vi "live view D04.vi"() -> ()   [LabVIEW 2019, in "D04.lvlib"]
uses:
  D04.lvlib
  <vilib>/userDefined/High Color/IMAQdx.ctl
  <vilib>/vision/Image Controls.llb/IMAQ Image.ctl
  <vilib>/measure/mamon.llb/Trigger Detection for 1 Channel.vi
  <vilib>/measure/NI_MAPro.lvlib
  Calibration Lib.lvlib
  database.lvlib
  <vilib>/vision/driver/NI_Vision_Acquisition_Software.lvlib
panel:
  out "Error out":errorcluster
  in  "Save Button":bool
  in  "Calib IMQ Num":u16(ring) items=["First IMQ", "Second IMQ", "Third IMQ"]
  in  "Verify Calibration1 D04":bool caption="capture grab"
  in  "snapshot":bool
  out "error prj03":errorcluster
  in  "Verify Calibration D04":bool caption="capture grab"
  in  "Close":bool
  in  "Method 2 save D04":bool caption="capture grab"
  in  "Method 1 Save D04":bool caption="Saving txt"
  out "Average Result":string="Average Result"
  out ">18  A":dbl(slide)=1.0 caption=">18 mm" scale=0.0..100.0
  out "16-18  A":dbl(slide)=1.0 caption="16-18 mm" scale=0.0..100.0
  out "14-16  A":dbl(slide)=1.0 caption="14-16 mm" scale=0.0..100.0
  out "12.5-14 A":dbl(slide)=1.0 caption="12.5-14 mm" scale=0.0..100.0
  out "10-12.5  A":dbl(slide)=1.0 caption="10-12.5 mm" scale=0.0..100.0 scale format="%#_4f"
  out "8-10  A":dbl(slide)=1.0 caption="8-10 mm" scale=0.0..100.0
  out "6.3-8  A":dbl(slide)=1.0 caption="6.3-8 mm" scale=0.0..100.0
  out "<6.3  A":dbl(slide)=1.0 caption="<6.3 mm" scale=0.0..100.0
  out "Live Result":string="Live Result"
  out ">18  L":dbl(slide)=1.0 caption=">18 mm" scale=0.0..100.0
  out "Live View":T1(plugin-control) caption="Disc 26"
  out "16-18  L":dbl(slide)=1.0 caption="16-18 mm" scale=0.0..100.0
  out "14-16  L":dbl(slide)=1.0 caption="14-16 mm" scale=0.0..100.0
  out "12.5-14 L":dbl(slide)=1.0 caption="12.5-14 mm" scale=0.0..100.0
  out "10-12.5  L":dbl(slide)=1.0 caption="10-12.5 mm" scale=0.0..100.0 scale format="%#_4f"
  out "8-10  L":dbl(slide)=1.0 caption="8-10 mm" scale=0.0..100.0
  out "6.3-8  L":dbl(slide)=1.0 caption="6.3-8 mm" scale=0.0..100.0
  out "<6.3  L":dbl(slide)=1.0 caption="<6.3 mm" scale=0.0..100.0
  out "disc name":string="Live Info Disc 04"
  out "dsgs":string="DSGS"
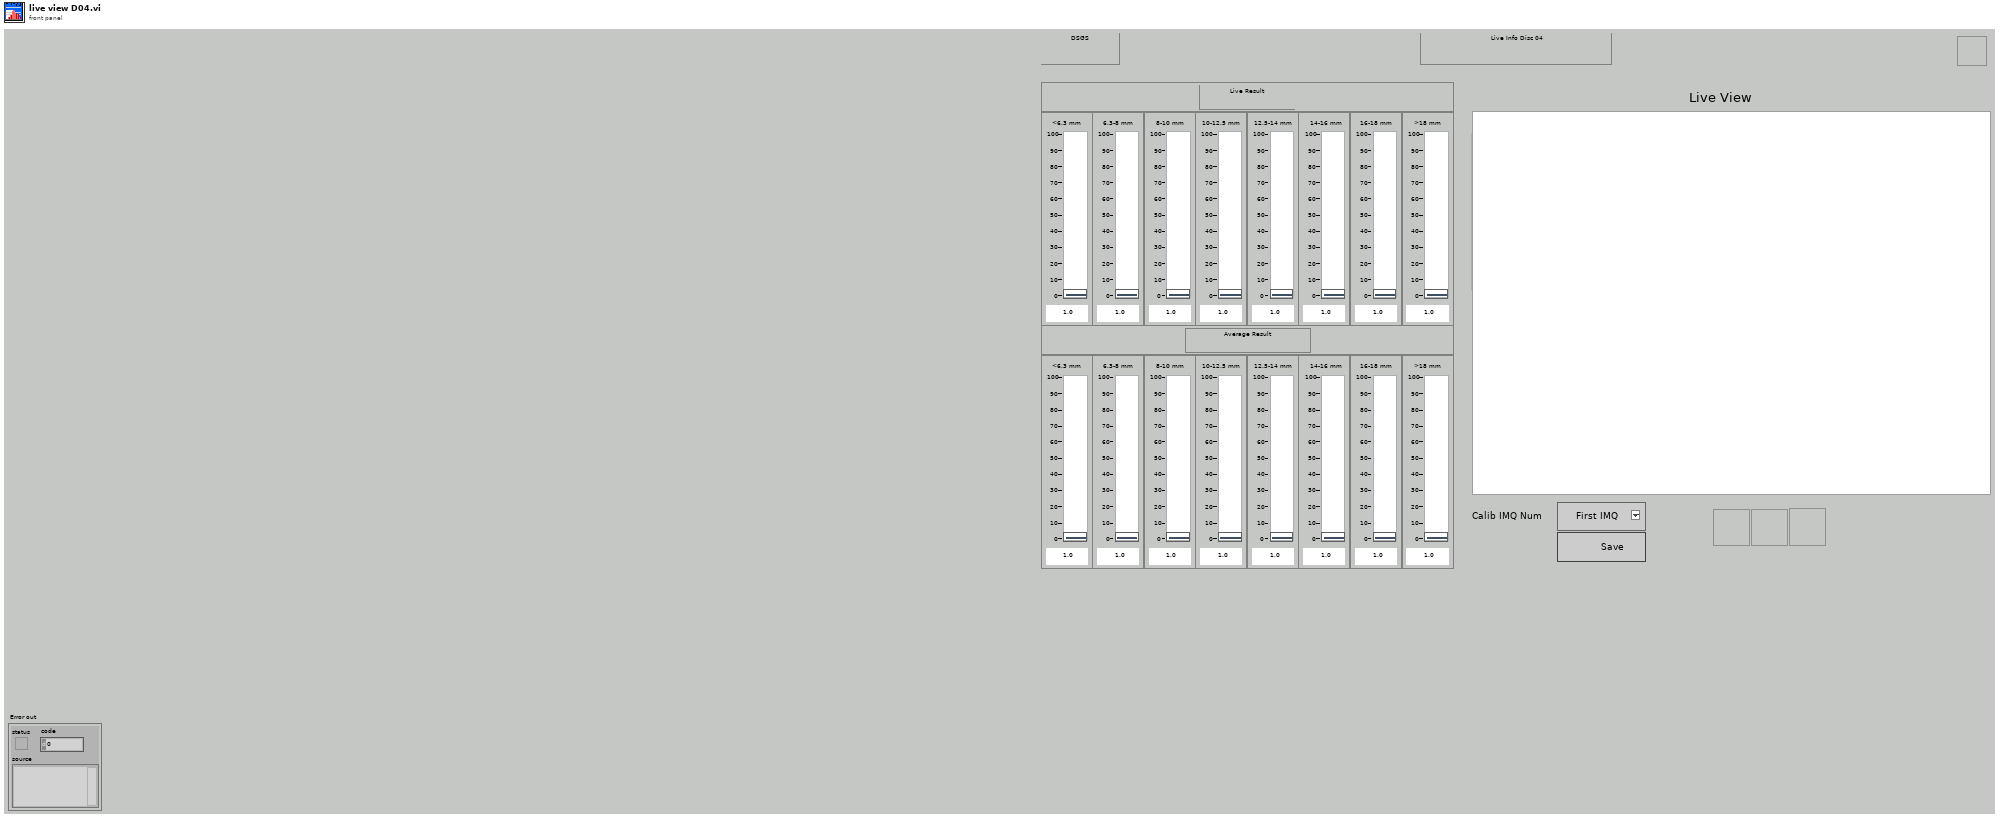
[diagram p1: front panel]
types:
  T1 = typedef "IMAQ Image.ctl" = refnum<image>
  T2 = typedef "IMAQdx.ctl" = refnum<k21>
  T3 = enum8{"Enabled", "Disabled", "Disabled and Grayed Out"}
  T4 = cluster{"date/time string":string, "date/time string":string, string, "Value":dbl, "Value":dbl, "Value":dbl, "Value":dbl, "Value":dbl, "Value":dbl, "Value":dbl, "Value":dbl}
  T5 = cluster{"date/time string":string, "date/time string":string, "time format string (%c)":string, "spreadsheet string":string, "spreadsheet string":string}
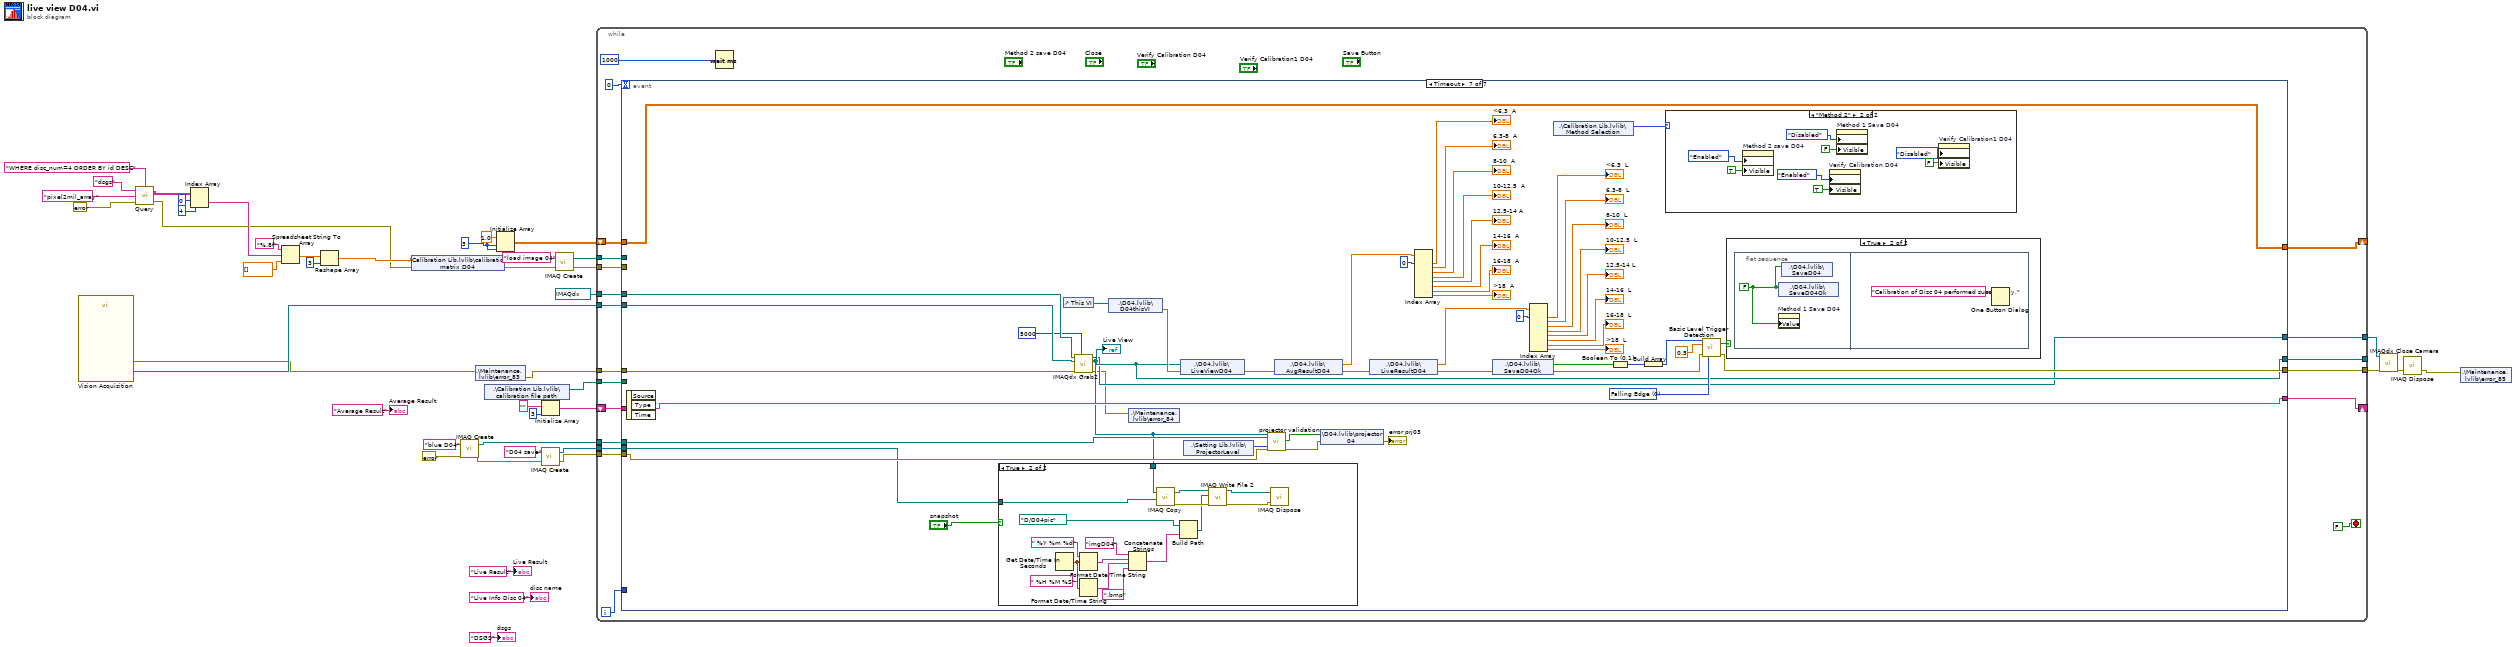
[diagram p0: block diagram]
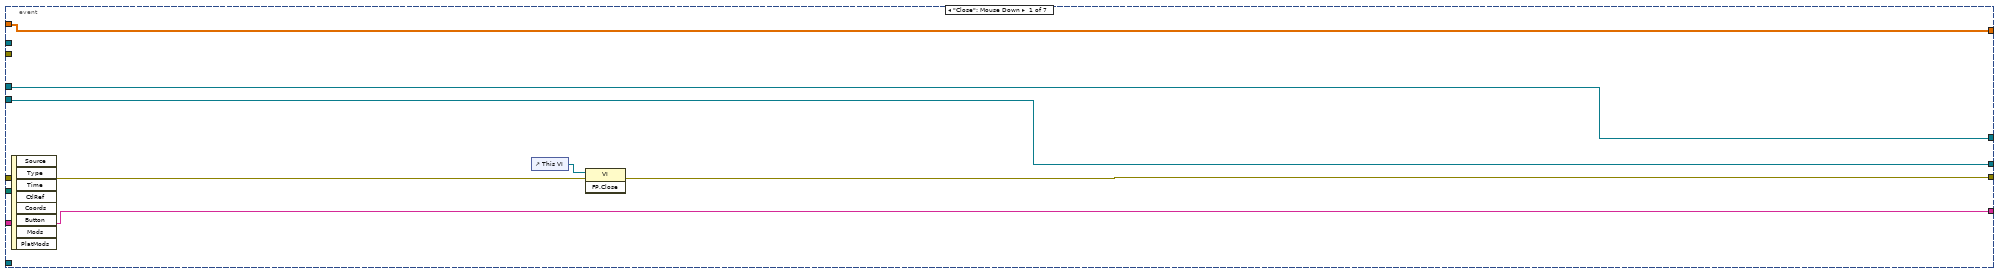
[diagram p2: hidden frame]
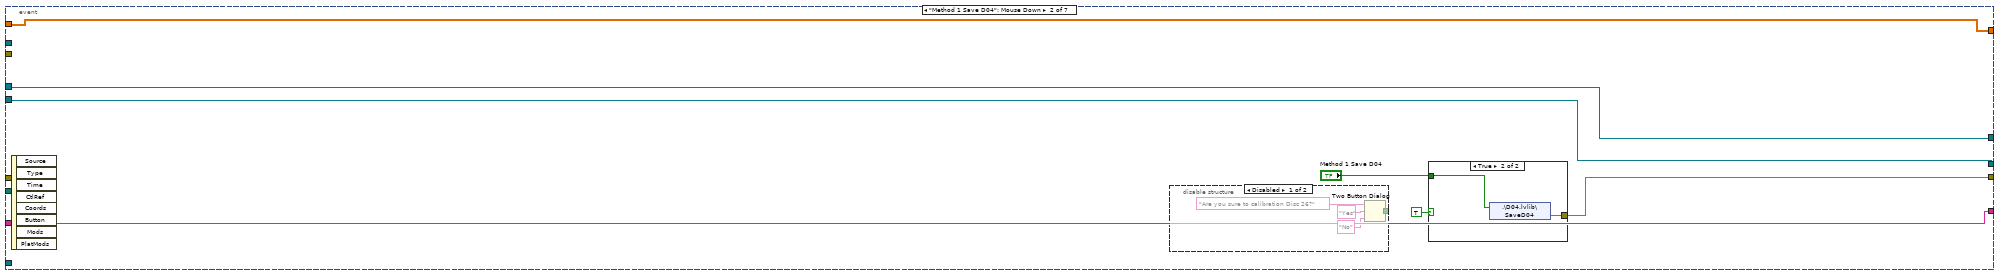
[diagram p3: hidden frame]
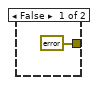
[diagram p5: hidden frame]
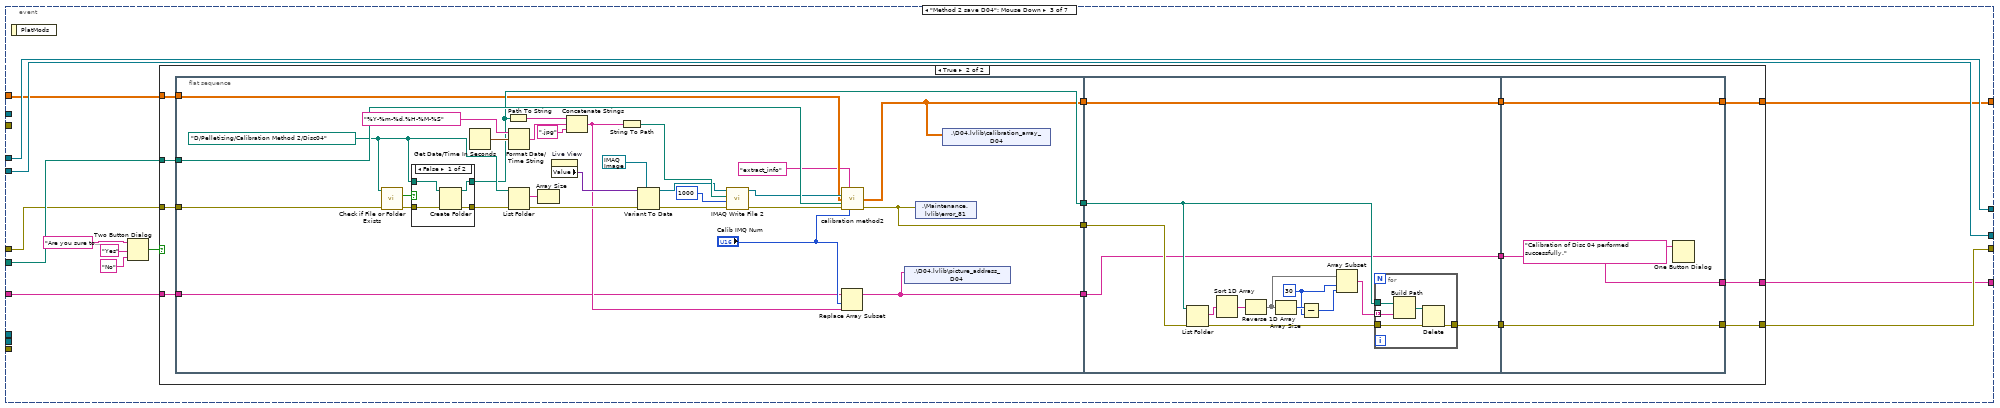
[diagram p6: hidden frame]
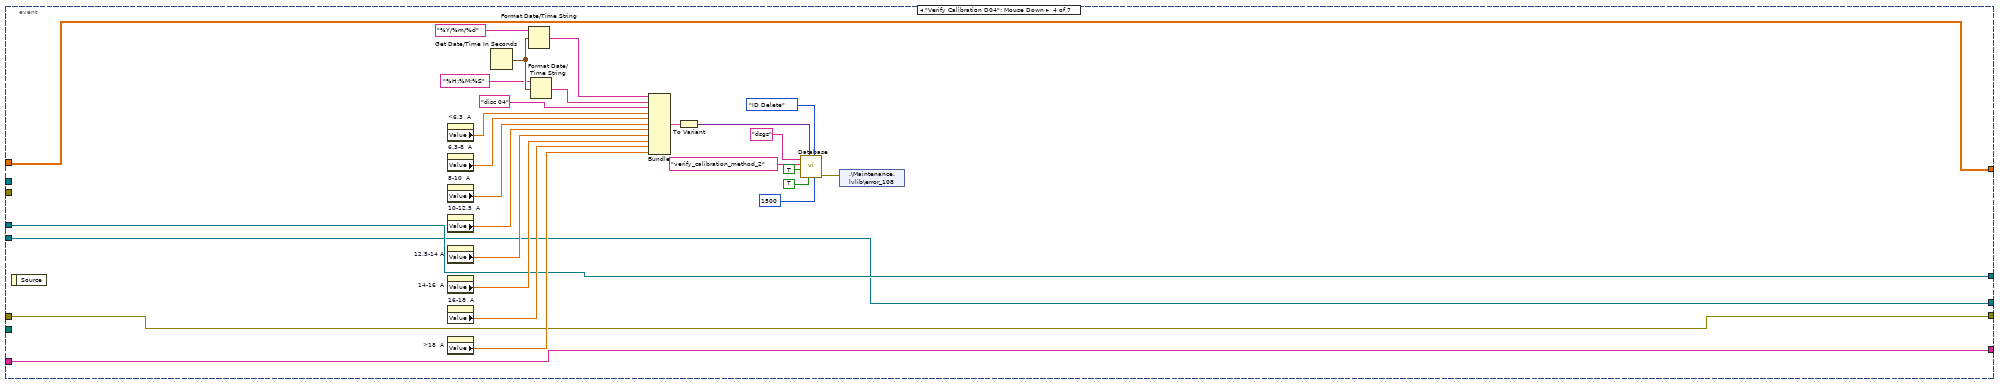
[diagram p9: hidden frame]
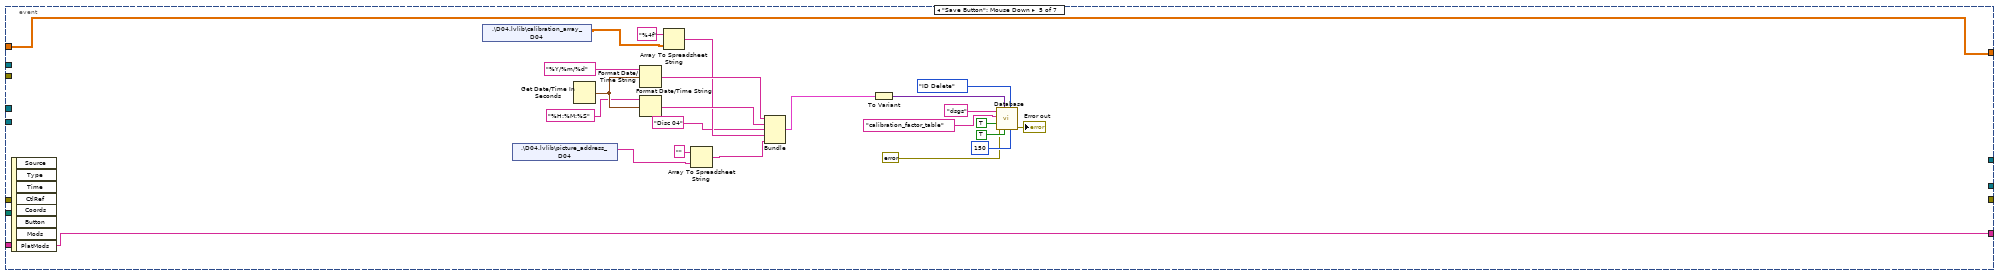
[diagram p10: hidden frame]
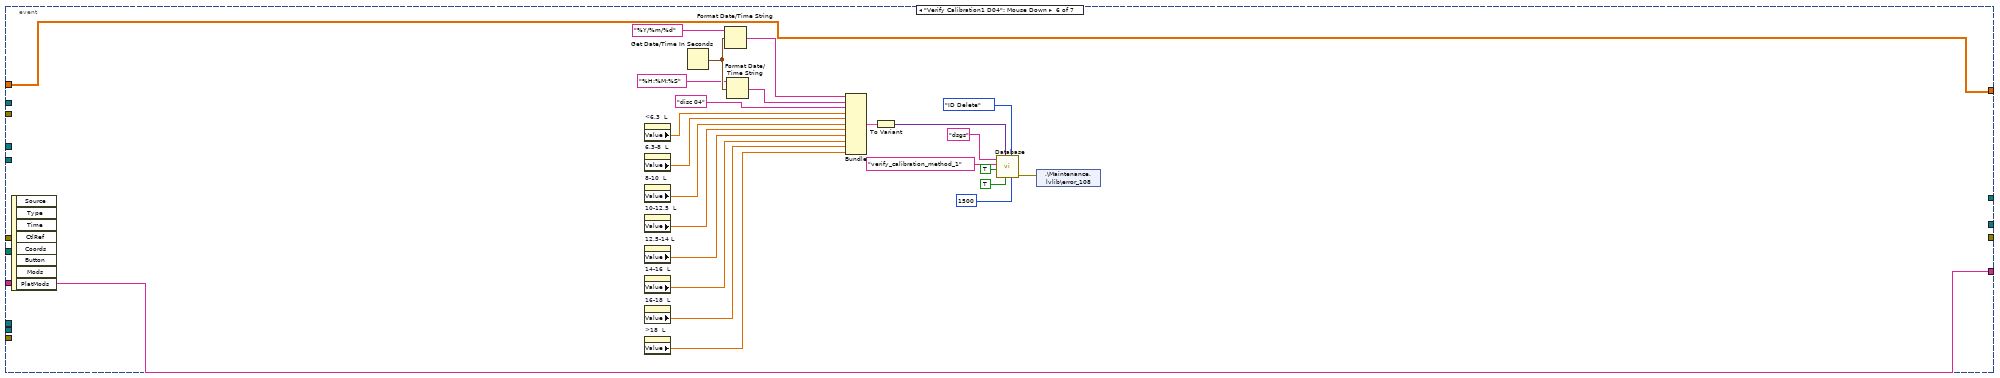
[diagram p11: hidden frame]
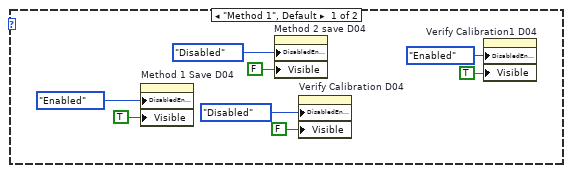
[diagram p13: hidden frame]
diagram:
  w13 = 3 ("dimension size")
  n1 = call "Vision Acquisition"() -> ("Image Out"=w2:T1, "error out"=w1:errorcluster)  [unwired: 25 in, 1 out]
  n2 = call "Query.vi"("Condition"="WHERE disc_num=4 ORDER BY id DESC", "Error in"=errorcluster {"status"=FALSE, "code"=0, "source"=""}, "Table Name"="pixel2mil_array", "Connection Name"="dsgs") -> ("Error out"=w5:errorcluster, "data"=w8:string[][])
  n3 = Index Array(array=w8, index (row)=0, index (col)=4 ("disabled index (col)")) -> (element=w6:string)
  n4 = Spreadsheet String To Array(format string="%.8f", spreadsheet string=w6, array type (2D Dbl)=sgl[] []) -> (array=w26:sgl[])  [unwired: 1 in]
  n5 = Reshape Array(w26, 3 ("dimension size")) -> (w23:sgl[])
  n6 = shared-variable ".\\Calibration Lib.lvlib\\calibration matrix D04"(w23, error in=w5) -> (error out=w22:errorcluster)
  n7 = call "IMAQ Create"("Image Name"="blue D04", "error in (no error)"=errorcluster {"status"=FALSE, "code"=0, "source"=""}) -> ("New Image"=w20:T1, "error out"=w18:errorcluster)  [unwired: 3 in]
  n8 = shared-variable ".\\Maintenance.lvlib\\error_83"(w1) -> (error out=w35:errorcluster)  [unwired: 1 in]
  n9 = shared-variable ".\\Calibration Lib.lvlib\\calibration file path"() -> (w36:path)  [unwired: 1 in, 1 out]
  n10 = Initialize Array(1.0 ("element"), w13, w13) -> (w12:dbl[][])
  n11 = call "IMAQ Create"("Image Name"="D04 save", "error in (no error)"=w18) -> ("New Image"=w15:T1, "error out"=w17:errorcluster)  [unwired: 3 in]
  n12 = Initialize Array("", 3 ("dimension size")) -> (w9:string[])
  n13 = call "IMAQ Create"("Image Name"="load image 04", "error in (no error)"=w22) -> ("New Image"=w32:T1, "error out"=w33:errorcluster)  [unwired: 3 in]
  n14 = while {
    tunnel: w36 -> [w62]
    tunnel: w35 -> [w61]
    tunnel: w2 -> [w59]
    tunnel: [w58] -> w40
    tunnel: [w57] -> _
    tunnel: T2 "disc01" ("Session In") -> [w56]
    tunnel: [w55] -> w37
    tunnel: w33 -> [w54]
    tunnel: w32 -> [w53]
    tunnel: w20 -> [w52]
    tunnel: w17 -> [w51]
    tunnel: w15 -> [w50]
    shift-right: [w47] -> _
    shift-left: w12 -> [w48]
    shift-right: [w45] -> _
    shift-left: w9 -> [w46]
    i -> [w49]
    stop <- FALSE stop-if-true
    n15 = event shown="[6] Timeout" {
      selector: _ -> [_ _ _ _ _ _ _]
      dyn-events: _ -> [_ _ _ _ _ _ _]
      timeout: 0 -> [_ _ _ _ _ _ _]
      tunnel: w62 -> [_ _ w98 _ _ _ _]
      tunnel: [w70 w78 w94 w180 _ _ w269] -> w58
      tunnel: w61 -> [w69 _ w97 w180 _ _ w254]
      tunnel: w59 -> [w68 w77 w96 w178 _ _ w253]
      tunnel: [w68 w77 w96 w178 _ _ w257] -> w57
      tunnel: w56 -> [w67 w76 w95 w179 _ _ w256]
      tunnel: [w67 w76 w95 w179 _ _ w255] -> w55
      tunnel: w54 -> [_ _ _ _ _ _ _]
      tunnel: w53 -> [_ _ _ _ _ _ _]
      tunnel: w52 -> [_ _ _ _ _ _ w267]
      tunnel: w51 -> [_ _ _ _ _ _ w263]
      tunnel: w50 -> [_ _ _ _ _ _ w260]
      tunnel: w49 -> [_ _ _ _ _ _ _]
      tunnel: w48 -> [w66 w73 w89 w175 w204 w227 w259]
      tunnel: [w66 w73 w88 w175 w204 w227 w259] -> w47
      tunnel: w46 -> [w65 w72 w87 w174 w203 w226 w258]
      tunnel: [w65 w72 w86 w174 w203 w226 w258] -> w45
      event "Close": Mouse Down {
        n16 = event-data() -> ()  [unwired: 1 in, 8 out]
        n17 = control-ref of="This VI"() -> (w71:refnum<vi>)
        n18 = invoke class="VI" method="FP.Close"(reference=w71, error in=w69) -> (error out=w70:errorcluster)  [unwired: 1 in, 2 out]
      }
      event "Method 1 Save D04": Mouse Down {
        n19 = event-data() -> ()  [unwired: 1 in, 8 out]
        n20 = disable-structure shown="Disabled" {
          disable-tunnel: [w79 _] -> _
          frame Disabled {
            n21 = Two Button Dialog(message="Are you sure to calibration Disc 26?", 1:"No" ("F button name (\"Cancel\")"), 2:"Yes" ("T button name (\"OK\")")) -> (T button?=w79:bool)
          }
          frame Enabled {
          }
        }
        n22 = case shown="True" TRUE {
          tunnel: [errorcluster {"status"=FALSE, "code"=0, "source"=""} ("error IO") w85] -> w78
          tunnel: "Method 1 Save D04" -> [_ w84]
          frame False {
          }
          frame True {
            n23 = shared-variable ".\\D04.lvlib\\SaveD04"(w84) -> (error out=w85:errorcluster)  [unwired: 1 in]
          }
        }
      }
      event "Method 2 save D04": Mouse Down {
        n24 = event-data() -> ()  [unwired: 1 in, 1 out]
        n25 = Two Button Dialog(message="Are you sure to calibration Disc 26?", 1:"No" ("F button name (\"Cancel\")"), 2:"Yes" ("T button name (\"OK\")")) -> (T button?=w90:bool)
        n26 = case shown="True" w90 {
          tunnel: w98 -> [_ w114]
          tunnel: w97 -> [w101 w113]
          tunnel: [w101 w112] -> w94
          tunnel: w89 -> [w100 w110]
          tunnel: [w100 w107] -> w88
          tunnel: w87 -> [w99 w106]
          tunnel: [w99 w103] -> w86
          frame False {
          }
          frame True {
            n27 = flat-sequence {
              tunnel: w113 -> [w134]
              tunnel: w114 -> [w145]
              tunnel: [w127] -> w115
              tunnel: w110 -> [w124]
              tunnel: [w123] -> w108
              tunnel: w106 -> [w118]
              tunnel: [w117] -> w104
              tunnel: [w116] -> w102
              tunnel: [w155] -> w111
              tunnel: [w153] -> w109
              tunnel: [w152] -> w105
              tunnel: w102 -> [w156]
              tunnel: w104 -> [w152]
              tunnel: w108 -> [w153]
              tunnel: w115 -> [w157]
              tunnel: [w173] -> w112
              tunnel: w111 -> [w173]
              tunnel: [w171] -> w107
              tunnel: w109 -> [w171]
              tunnel: [w170] -> w103
              tunnel: w105 -> [w170]
              frame #0 {
                w128 = path "D:/Pelletizing/Calibration Method 2/Disc04" ("path")
                n28 = call <vilib>:"Check if File or Folder Exists.vi"("error in (no error)"=w134, "path"=w128) -> ("error out"=w135:errorcluster, "file or folder exists?"=w136:bool)  [unwired: 7 in, 1 out]
                n29 = case shown="False" w136 {
                  tunnel: [w147 w151] -> w127
                  tunnel: w128 -> [w149 w151]
                  tunnel: w135 -> [w148 w150]
                  tunnel: [w146 w150] -> w130
                  frame False {
                    n30 = Create Folder(path (use dialog)=w149, error in=w148) -> (created path=w147:path, error out=w146:errorcluster)  [unwired: 1 in, 1 out]
                  }
                  frame True {
                  }
                }
                n31 = Get Date/Time In Seconds() -> (seconds since 1Jan1904=w140:timestamp)
                n32 = Path To String(path=w127) -> (string=w132:string)
                n33 = Format Date/Time String(time format string (%c)="%Y-%m-%d,%H-%M-%S", seconds (now)=w140) -> (date/time string=w138:string)  [unwired: 1 in]
                n34 = List Folder(path=w128, error in=w130) -> (filenames=w131:string[], error out=w129:errorcluster)  [unwired: 2 in, 2 out]
                n35 = Array Size(array=w131) -> ()  [unwired: 1 out]
                n36 = property on="Live View" class="ImageControl"() -> ("Value"=w144:variant)  [unwired: 2 in, 2 out]
                n37 = Concatenate Strings(w132, w138, ".jpg" ("string")) -> (w120:string)
                n38 = String To Path(string=w120) -> (path=w133:path)
                n39 = Variant To Data(error in=w129, type=T1 refnum ("New Image"), Variant=w144) -> (data=w125:T1, error out=w141:errorcluster)
                n40 = call-poly "IMAQ Write File 2"("error in (no error)"=w141, "Image Quality"=u32 1000, "File Path"=w133, "Image"=w125) -> ("error out"=w122:errorcluster, "Image Out (duplicate)"=w126:T1)  [unwired: 6 in]
                n41 = Replace Array Subset(array=w118, new element=w120, index="Calib IMQ Num") -> (w117:string[])
                n42 = call "calibration method2.vi"("function name"="extract_info", "Image IN"=w126, "initialize matrix"=w124, "module path"=w145, "error in"=w122, "snap number"="Calib IMQ Num") -> ("calibration matrix"=w123:dbl[][], "error out"=w116:errorcluster)  [unwired: 8 in]
                n43 = shared-variable ".\\D04.lvlib\\picture_address_D04"(w117) -> ()  [unwired: 1 in, 1 out]
                n44 = shared-variable ".\\Maintenance.lvlib\\error_81"(w116) -> ()  [unwired: 1 in, 1 out]
                n45 = shared-variable ".\\D04.lvlib\\calibration_array_D04"(w123) -> ()  [unwired: 1 in, 1 out]
              }
              frame #1 {
                w158 = 30 ("index")
                n46 = List Folder(path=w157, error in=w156) -> (filenames=w164:string[], error out=w154:errorcluster)  [unwired: 2 in, 2 out]
                n47 = Sort 1D Array(array=w164) -> (sorted array=w163:string[])
                n48 = Reverse 1D Array(array=w163) -> (reversed array=w162:string[])
                n49 = Array Size(array=w162) -> (size(s)=w161:i32)
                n50 = Subtract(x=w161, y=w158) -> (x-y=w160:i32)
                n51 = Array Subset(array=w162, index=w158, length=w160) -> (w159:string[])
                n52 = for {
                  tunnel: w159 -> [w168] mode=indexing
                  tunnel: w157 -> [w169]
                  tunnel: [w166] -> w155
                  tunnel: w154 -> [w165]
                  n53 = Build Path(base path=w169, name or relative path=w168) -> (appended path=w167:path)
                  n54 = Delete(path (use dialog)=w167, error in=w165) -> (error out=w166:errorcluster)  [unwired: 3 in, 2 out]
                }
              }
              frame #2 {
                n55 = One Button Dialog(message="Calibration of Disc 04 performed successfully.") -> ()  [unwired: 1 in, 1 out]
              }
            }
          }
        }
      }
      event "Verify Calibration D04": Mouse Down {
        n56 = event-data() -> ()  [unwired: 1 in, 1 out]
        n57 = property on="<6.3  A" class="Slide (strict)"() -> ("Value"=w195:dbl)  [unwired: 2 in, 2 out]
        n58 = property on="6.3-8  A" class="Slide (strict)"() -> ("Value"=w194:dbl)  [unwired: 2 in, 2 out]
        n59 = property on="8-10  A" class="Slide (strict)"() -> ("Value"=w193:dbl)  [unwired: 2 in, 2 out]
        n60 = property on="10-12.5  A" class="Slide (strict)"() -> ("Value"=w192:dbl)  [unwired: 2 in, 2 out]
        n61 = property on="12.5-14 A" class="Slide (strict)"() -> ("Value"=w191:dbl)  [unwired: 2 in, 2 out]
        n62 = property on="14-16  A" class="Slide (strict)"() -> ("Value"=w190:dbl)  [unwired: 2 in, 2 out]
        n63 = property on="16-18  A" class="Slide (strict)"() -> ("Value"=w189:dbl)  [unwired: 2 in, 2 out]
        n64 = property on=">18  A" class="Slide (strict)"() -> ("Value"=w188:dbl)  [unwired: 2 in, 2 out]
        n65 = Get Date/Time In Seconds() -> (seconds since 1Jan1904=w200:timestamp)
        n66 = Format Date/Time String(time format string (%c)="%Y/%m/%d", seconds (now)=w200) -> (date/time string=w198:string)  [unwired: 1 in]
        n67 = Format Date/Time String(time format string (%c)="%H:%M:%S", seconds (now)=w200) -> (date/time string=w197:string)  [unwired: 1 in]
        n68 = Bundle("date/time string"=w198, "date/time string"=w197, "disc 04", "Value"=w195, "Value"=w194, "Value"=w193, "Value"=w192, "Value"=w191, "Value"=w190, "Value"=w189, "Value"=w188) -> (w187:T4)  [unwired: 1 in]
        n69 = To Variant(anything=w187) -> (Variant=w186:variant)
        n70 = call "Database.vi"("Maximum Row"=1500, "Enum"=enum16{"ID Delete", "Time Delete"}."ID Delete", "Delete row?"=TRUE, "Data"=w186, "Auto Increment ID?"=TRUE, "Table"="verify_calibration_method_2", "Connection"="dsgs") -> ("Error out"=w181:errorcluster)  [unwired: 4 in]
        n71 = shared-variable ".\\Maintenance.lvlib\\error_108"(w181) -> ()  [unwired: 1 in, 1 out]
      }
      event "Save Button": Mouse Down {
        n72 = event-data() -> ()  [unwired: 1 in, 8 out]
        n73 = shared-variable ".\\D04.lvlib\\calibration_array_D04"() -> (w205:dbl[][])  [unwired: 1 in, 1 out]
        n74 = shared-variable ".\\D04.lvlib\\picture_address_D04"() -> (w207:string[])  [unwired: 1 in, 1 out]
        n75 = Get Date/Time In Seconds() -> (seconds since 1Jan1904=w214:timestamp)
        n76 = Format Date/Time String(time format string (%c)="%Y/%m/%d", seconds (now)=w214) -> (date/time string=w215:string)  [unwired: 1 in]
        n77 = Format Date/Time String(time format string (%c)="%H:%M:%S", seconds (now)=w214) -> (date/time string=w213:string)  [unwired: 1 in]
        n78 = Array To Spreadsheet String(array=w205, 3:"%4f" ("format string")) -> (spreadsheet string=w209:string)  [unwired: 1 in]
        n79 = Array To Spreadsheet String(array=w207, 3:"" ("format string")) -> (spreadsheet string=w206:string)  [unwired: 1 in]
        n80 = Bundle("date/time string"=w215, "date/time string"=w213, "time format string (%c)"="Disc 04", "spreadsheet string"=w209, "spreadsheet string"=w206) -> (w218:T5)  [unwired: 1 in]
        n81 = To Variant(anything=w218) -> (Variant=w225:variant)
        n82 = call "Database.vi"("Maximum Row"=150, "Enum"=enum16{"ID Delete", "Time Delete"}."ID Delete", "Delete row?"=TRUE, "Data"=w225, "Error in"=errorcluster {"status"=FALSE, "code"=0, "source"=""}, "Auto Increment ID?"=TRUE, "Table"="calibration_factor_table", "Connection"="dsgs") -> ("Error out"=→"Error out":errorcluster)  [unwired: 3 in]
      }
      event "Verify Calibration1 D04": Mouse Down {
        n83 = event-data() -> ()  [unwired: 1 in, 8 out]
        n84 = property on="<6.3  L" class="Slide (strict)"() -> ("Value"=w244:dbl)  [unwired: 2 in, 2 out]
        n85 = property on="6.3-8  L" class="Slide (strict)"() -> ("Value"=w243:dbl)  [unwired: 2 in, 2 out]
        n86 = property on="8-10  L" class="Slide (strict)"() -> ("Value"=w242:dbl)  [unwired: 2 in, 2 out]
        n87 = property on="10-12.5  L" class="Slide (strict)"() -> ("Value"=w241:dbl)  [unwired: 2 in, 2 out]
        n88 = property on="12.5-14 L" class="Slide (strict)"() -> ("Value"=w240:dbl)  [unwired: 2 in, 2 out]
        n89 = property on="14-16  L" class="Slide (strict)"() -> ("Value"=w239:dbl)  [unwired: 2 in, 2 out]
        n90 = property on="16-18  L" class="Slide (strict)"() -> ("Value"=w238:dbl)  [unwired: 2 in, 2 out]
        n91 = property on=">18  L" class="Slide (strict)"() -> ("Value"=w237:dbl)  [unwired: 2 in, 2 out]
        n92 = Get Date/Time In Seconds() -> (seconds since 1Jan1904=w249:timestamp)
        n93 = Format Date/Time String(time format string (%c)="%Y/%m/%d", seconds (now)=w249) -> (date/time string=w247:string)  [unwired: 1 in]
        n94 = Format Date/Time String(time format string (%c)="%H:%M:%S", seconds (now)=w249) -> (date/time string=w246:string)  [unwired: 1 in]
        n95 = Bundle("date/time string"=w247, "date/time string"=w246, "disc 04", "Value"=w244, "Value"=w243, "Value"=w242, "Value"=w241, "Value"=w240, "Value"=w239, "Value"=w238, "Value"=w237) -> (w236:T4)  [unwired: 1 in]
        n96 = To Variant(anything=w236) -> (Variant=w235:variant)
        n97 = call "Database.vi"("Maximum Row"=1500, "Enum"=enum16{"ID Delete", "Time Delete"}."ID Delete", "Delete row?"=TRUE, "Data"=w235, "Auto Increment ID?"=TRUE, "Table"="verify_calibration_method_1", "Connection"="dsgs") -> ("Error out"=w230:errorcluster)  [unwired: 4 in]
        n98 = shared-variable ".\\Maintenance.lvlib\\error_108"(w230) -> ()  [unwired: 1 in, 1 out]
      }
      event Timeout {
        w277 = u16 0 items=["Falling Edge", "Rising Edge"] ("trigger slope")
        n99 = event-data() -> ()  [unwired: 1 in, 3 out]
        n100 = control-ref of="This VI"() -> (w272:refnum<vi>)
        n101 = call <vilib>:"IMAQdx Grab2.vi"("Timeout (ms)"=5000, "error in"=w254, "Image In"=w253, "Session In"=w256) -> ("error out"=w251:errorcluster, "Image Out"=w257:T1, "Session Out"=w255:T2)  [unwired: 4 in, 1 out]
        "Live View" <- w257
        n102 = case shown="True" "snapshot" {
          tunnel: w260 -> [_ w317]
          tunnel: w257 -> [_ w316]
          frame False {
          }
          frame True {
            n103 = Get Date/Time In Seconds() -> (seconds since 1Jan1904=w310:timestamp)
            n104 = Format Date/Time String(time format string (%c)=" %Y %m %d", seconds (now)=w310) -> (date/time string=w306:string)  [unwired: 1 in]
            n105 = Format Date/Time String(time format string (%c)=" %H %M %S", seconds (now)=w310) -> (date/time string=w305:string)  [unwired: 1 in]
            n106 = Concatenate Strings("imgD04" ("string"), w306, w305, ".bmp" ("string")) -> (w303:string)
            n107 = call "IMAQ Copy"("Image Dst"=w317, "Image Src"=w316) -> ("error out"=w314:errorcluster, "Image Dst Out"=w315:T1)  [unwired: 4 in]
            n108 = Build Path(base path=path "D:/D04pic" ("File Path"), name or relative path=w303) -> (appended path=w302:path)
            n109 = call-poly "IMAQ Write File 2"("error in (no error)"=w314, "File Path"=w302, "Image"=w315) -> ("error out"=w312:errorcluster, "Image Out (duplicate)"=w313:T1)  [unwired: 7 in]
            n110 = call "IMAQ Dispose"("Image"=w313, "error in (no error)"=w312) -> ()  [unwired: 4 in, 1 out]
          }
        }
        n111 = shared-variable ".\\D04.lvlib\\D04thisVI"(w272) -> (error out=w268:errorcluster)  [unwired: 1 in]
        n112 = shared-variable ".\\Maintenance.lvlib\\error_84"(w251) -> ()  [unwired: 1 in, 1 out]
        n113 = shared-variable ".\\D04.lvlib\\LiveViewD04"(w257, error in=w268) -> (error out=w271:errorcluster)
        n114 = shared-variable ".\\Setting Lib.lvlib\\ProjectorLevel"() -> (w262:i32)  [unwired: 1 in, 1 out]
        n115 = call "projector validation.vi"("Image Src"=w257, "blue channel"=w267, "on/off level"=w262, "error in (no error)"=w263) -> ("on/off"=w266:bool, "error out"=w265:errorcluster)  [unwired: 14 in]
        n116 = shared-variable ".\\D04.lvlib\\AvgResultD04"(error in=w271) -> (w292:dbl[], error out=w274:errorcluster)
        n117 = shared-variable ".\\D04.lvlib\\projector 04"(w266, error in=w265) -> (error out=→"error prj03":errorcluster)
        n118 = shared-variable ".\\D04.lvlib\\LiveResultD04"(error in=w274) -> (w291:dbl[], error out=w273:errorcluster)
        n119 = Index Array(array=w292, index #1=0 ("index")) -> (element #1=→"<6.3  A":dbl, element #2=→"6.3-8  A":dbl, element #3=→"8-10  A":dbl, element #4=→"10-12.5  A":dbl, element #5=→"12.5-14 A":dbl, element #6=→"14-16  A":dbl, element #7=→"16-18  A":dbl, element #8=→">18  A":dbl)  [unwired: 7 in]
        n120 = shared-variable ".\\D04.lvlib\\SaveD04Ok"(error in=w273) -> (w278:bool, error out=w270:errorcluster)
        n121 = Index Array(array=w291, index #1=0 ("index")) -> (element #1=→"<6.3  L":dbl, element #2=→"6.3-8  L":dbl, element #3=→"8-10  L":dbl, element #4=→"10-12.5  L":dbl, element #5=→"12.5-14 L":dbl, element #6=→"14-16  L":dbl, element #7=→"16-18  L":dbl, element #8=→">18  L":dbl)  [unwired: 7 in]
        n122 = shared-variable ".\\Calibration Lib.lvlib\\Method Selection"() -> (w275:enum32{"Method 1", "Method 2"})  [unwired: 1 in, 1 out]
        n123 = Boolean To (0,1)(Boolean=w278) -> (0, 1=w281:i16)
        n124 = Build Array(w281) -> (w280:i16[])
        n125 = case shown="\"Method 2\"" w275 {
          frame "Method 1", Default {
            n126 = property on="Method 1 Save D04" class="Bool (strict)"("DisabledEnum"=T3."Enabled" ("Disabled"), "Visible"=TRUE) -> ()  [unwired: 2 in, 2 out]
            n127 = property on="Method 2 save D04" class="Bool (strict)"("DisabledEnum"=T3."Disabled" ("Disabled"), "Visible"=FALSE) -> ()  [unwired: 2 in, 2 out]
            n128 = property on="Verify Calibration D04" class="Bool (strict)"("DisabledEnum"=T3."Disabled" ("Disabled"), "Visible"=FALSE) -> ()  [unwired: 2 in, 2 out]
            n129 = property on="Verify Calibration1 D04" class="Bool (strict)"("DisabledEnum"=T3."Enabled" ("Disabled"), "Visible"=TRUE) -> ()  [unwired: 2 in, 2 out]
          }
          frame "Method 2" {
            n130 = property on="Method 2 save D04" class="Bool (strict)"("DisabledEnum"=T3."Enabled" ("Disabled"), "Visible"=TRUE) -> ()  [unwired: 2 in, 2 out]
            n131 = property on="Verify Calibration D04" class="Bool (strict)"("DisabledEnum"=T3."Enabled" ("Disabled"), "Visible"=TRUE) -> ()  [unwired: 2 in, 2 out]
            n132 = property on="Method 1 Save D04" class="Bool (strict)"("DisabledEnum"=T3."Disabled" ("Disabled"), "Visible"=FALSE) -> ()  [unwired: 2 in, 2 out]
            n133 = property on="Verify Calibration1 D04" class="Bool (strict)"("DisabledEnum"=T3."Disabled" ("Disabled"), "Visible"=FALSE) -> ()  [unwired: 2 in, 2 out]
          }
        }
        n134 = call-poly <vilib>:"Basic Level Trigger Detection.vi"("signal in"=w280, "level"=0.5, "error in (no error)"=w270, "trigger slope"=w277) -> ("trigger detected?"=w276:bool, "error out"=w269:errorcluster)  [unwired: 9 in, 1 out]
        n135 = case shown="True" w276 {
          frame False {
          }
          frame True {
            n136 = flat-sequence {
              frame #0 {
                w334 = FALSE
                n137 = shared-variable ".\\D04.lvlib\\SaveD04Ok"(w334) -> ()  [unwired: 1 in, 1 out]
                n138 = property on="Method 1 Save D04" class="Bool (strict)"("Value"=w334) -> ()  [unwired: 2 in, 2 out]
                n139 = shared-variable ".\\D04.lvlib\\SaveD04"(w334) -> ()  [unwired: 1 in, 1 out]
              }
              frame #1 {
                n140 = One Button Dialog(message="Calibration of Disc 04 performed successfully.") -> ()  [unwired: 1 in, 1 out]
              }
            }
          }
        }
      }
    }
    n141 = Wait (ms)(milliseconds to wait=u32 1000) -> ()  [unwired: 1 out]
  }
  n142 = call <vilib>:"IMAQdx Close Camera.vi"("error in"=w40, "Session In"=w37) -> ("error out"=w39:errorcluster)  [unwired: 9 in]
  n143 = call "IMAQ Dispose"("error in (no error)"=w39) -> ("error out"=w3:errorcluster)  [unwired: 5 in]
  n144 = shared-variable ".\\Maintenance.lvlib\\error_85"(w3) -> ()  [unwired: 1 in, 1 out]
  "Live Result" <- "Live Result" ("Live Result")
  "Average Result" <- "Average Result" ("Average Result")
  "disc name" <- "Live Info Disc 04" ("Live Result")
  "dsgs" <- "DSGS" ("Live Result")
